vi "image2bits_2.vi"(3 "Packet\nMessage Length (bits)":i32, 5 "path to JPEG file":path) -> (0 "Number of Packets":i32, 1 "Bitstream with Guard":u8[](array[numeric]), 2 "Transmitted picture":picture)   [LabVIEW 2019]
uses:
  <vilib>/picture/picture.llb/Draw True-Color Pixmap.vi
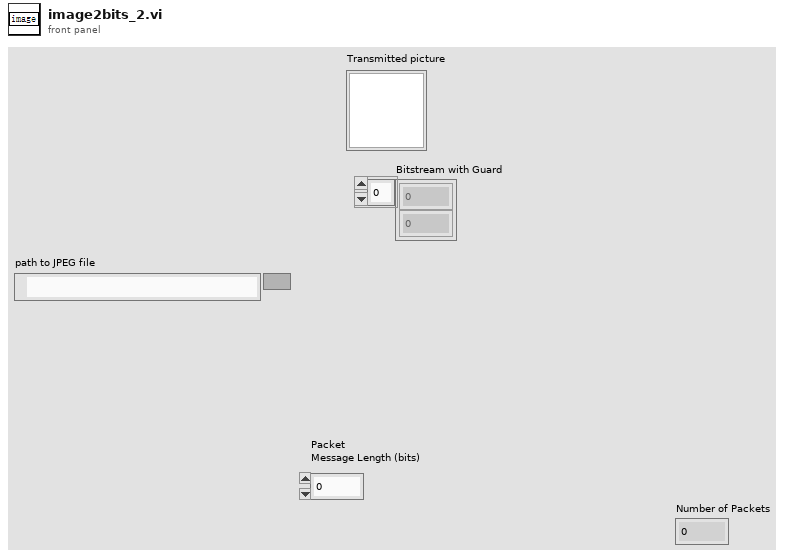
[diagram p1: front panel]
types:
  T1 = typedef "imagedata.ctl" = cluster{"image type":i32, "image depth":i32, "image":u8[], "mask":u8[], "colors":u32[], "Rectangle":cluster{"left":i16, "top":i16, "right":i16, "bottom":i16}}
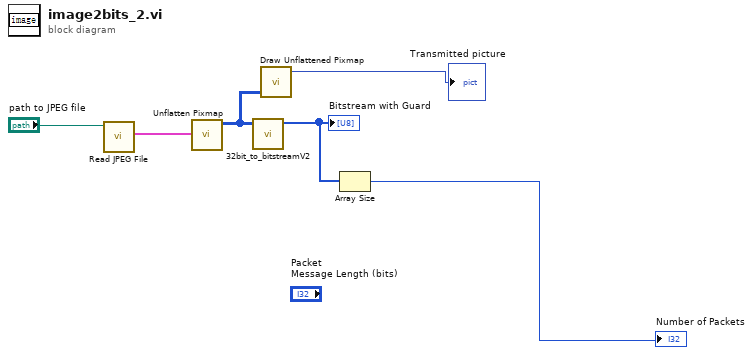
[diagram p0: block diagram]
diagram:
  n1 = call <vilib>:"Read JPEG File.vi"("path to JPEG file"="path to JPEG file") -> ("image data"=w5:T1)  [unwired: 8 in, 2 out]
  n2 = call <vilib>:"Unflatten Pixmap.vi"("image data"=w5) -> ("24-bit pixmap"=w4:u32[][])  [unwired: 4 in, 6 out]
  n3 = call "32bit_to_bitstreamV2.vi"("24-bit pixmap"=w4) -> ("Bitstream with Guard"=w2:u8[])  [unwired: 7 in, 1 out]
  "Bitstream with Guard" <- w2
  n4 = call-poly <vilib>:"Draw Unflattened Pixmap.vi"("data (RGB format)"=w4) -> ("new picture"=→"Transmitted picture":picture)  [unwired: 8 in]
  n5 = Array Size(array=w2) -> (size(s)=→"Number of Packets":i32)
